vi "Load Cfg.vi"(8 "error in (no error)":errorcluster, 11 "Socket in":refnum<class "Socket.lvclass">) -> (0 "error out":errorcluster, 3 "Socket out":refnum<class "Socket.lvclass">)   [LabVIEW 2018, in "Socket.lvclass"]
uses:
  Socket.lvclass
  Socket.lvclass/Socket.ctl
  <vilib>/Utility/config.llb/Read Key (String).vi
  <vilib>/Utility/config.llb/Read Key (Boolean).vi
  <vilib>/Utility/config.llb/NI_LVConfig.lvlib
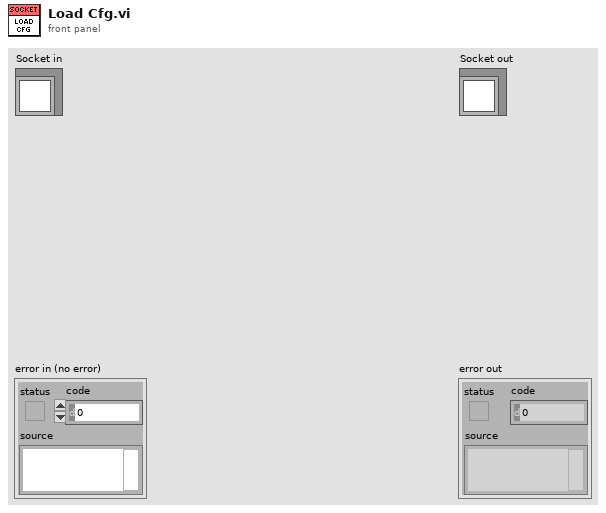
[diagram p1: front panel]
types:
  T1 = typedef "NI_LVConfig.lvlib/Config Data RefNum.ctl" = refnum<k1>
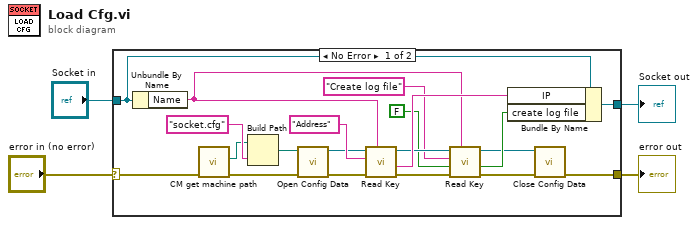
[diagram p0: block diagram]
diagram:
  n1 = case shown="No Error" "error in (no error)" {
    selector: "error in (no error)" -> [w16 w26]
    tunnel: [w15 w26] -> w3
    tunnel: [w13 w25] -> w1
    tunnel: "Socket in" -> [w17 w25]
    frame No Error {
      n2 = Unbundle By Name(w17) -> ("Name"=w10:string)
      n3 = call "CM get machine path.vi"("error in (no error) 2"=w16) -> ("error in (no error)"=w18:errorcluster, "machine path"=w19:path)  [unwired: 9 in]
      n4 = Build Path(base path=w19, name or relative path="socket.cfg") -> (appended path=w24:path)
      n5 = call <vilib>:"Open Config Data.vi"("error in (no error)"=w18, "configuration file path"=w24) -> ("error out"=w20:errorcluster, "refnum"=w21:T1)  [unwired: 7 in, 1 out]
      n6 = call-poly <vilib>:"Read Key.vi"("section"=w10, "error in (no error)"=w20, "key"="Address", "refnum"=w21) -> ("error out"=w12:errorcluster, "value"=w14:string, "refnum out"=w8:T1)  [unwired: 4 in, 1 out]
      n7 = call-poly <vilib>:"Read Key.vi"("section"=w10, "error in (no error)"=w12, "default value"=FALSE, "key"="Create log file", "refnum"=w8) -> ("error out"=w11:errorcluster, "value"=w9:bool, "refnum out"=w7:T1)  [unwired: 3 in, 1 out]
      n8 = Bundle By Name(cluster=w17, "IP"=w14, "create log file"=w9) -> (w13:refnum<class "Socket.lvclass">)
      n9 = call <vilib>:"Close Config Data.vi"("error in (no error)"=w11, "refnum"=w7) -> ("error out"=w15:errorcluster)  [unwired: 8 in, 1 out]
    }
    frame Error {
    }
  }
  "error out" <- w3
  "Socket out" <- w1
